vi "Check Message Queue Status.vi"(0 "message queue in":T1, 11 "error in":errorcluster) -> (2 "max queue size":i32, 3 "message queue name":string, 4 "message queue out":T1, 6 "# elements in queue":i32, 15 "error out":errorcluster)   [LabVIEW 2013, in "AMC.lvlib"]
doc: "Returns the max queue size, message queue name, and the number of elements in the queue."
uses:
  AMC.lvlib
  Message Queue.ctl
  Message.ctl
  <vilib>/NI/Tools/Keyed Array/KeyedArray.ctl
  <vilib>/NI/Tools/Keyed Array/Tools_KeyedArray.lvlib
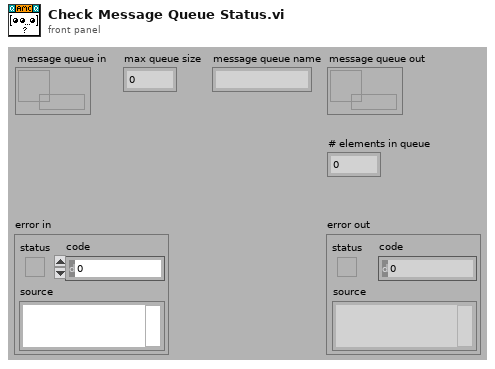
[diagram p1: front panel]
types:
  T1 = typedef "AMC.lvlib/Message Queue.ctl" = refnum<queue>
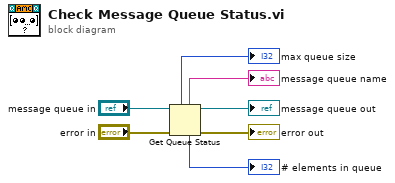
[diagram p0: block diagram]
diagram:
  n1 = Get Queue Status(queue="message queue in", error in (no error)="error in") -> (queue out=→"message queue out":T1, queue name=→"message queue name":string, max queue size=→"max queue size":i32, error out=→"error out":errorcluster, # elements in queue=→"# elements in queue":i32)  [unwired: 4 out]
